vi "Main - Auto Detect Modules.vi"(8 "error in (no error)":errorcluster, 11 "Node Ptr":u64 format="%.0x") -> (0 "error out":errorcluster)   [LabVIEW 2017, in "Scan Engine Custom Device.lvlib"]
uses:
  Scan Engine Custom Device.lvlib
  <vilib>/NI Veristand/Custom Device API/Custom Device Channel.ctl
  <vilib>/NI Veristand/Custom Device API/Custom Device Channel Type.ctl
  Modules.lvlibp/RSI Module/Slot Settings.ctl
  Modules.lvlibp/RSI Module/Module Models.ctl
  Type Defs/Host - FPGAScanInterfaceMode.ctl
  Globals/String Constants.vi
  Globals/Scan Engine GUIDs.vi
  Globals/Property Strings.vi
  <vilib>/NI Veristand/Custom Device API/Set Item Property (String).vi
  Modules.lvlibp/RSI Module/Class Property Strings.vi
  Modules.lvlibp/RSI Module/RSI Module.lvclass
  Modules.lvlibp/RemIO Module/RemIO Module.lvclass
  <vilib>/NI Veristand/Custom Device API/Custom Device API.lvlib
  Modules.lvlibp
  <resource>/objmgr/ni.var.rc
panel:
  in  "Tag":string
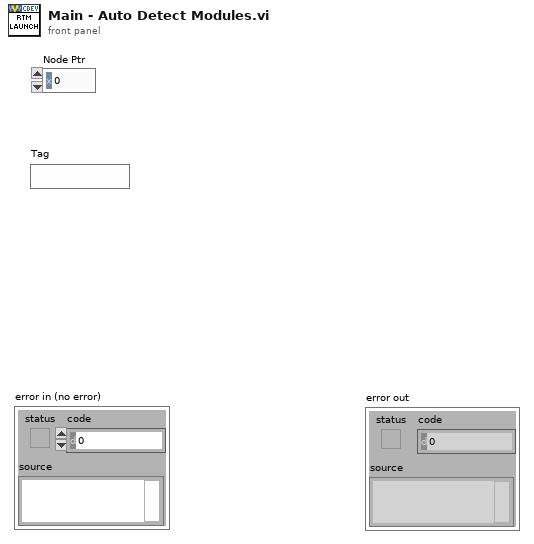
[diagram p1: front panel]
types:
  T1 = typedef "Custom Device API.lvlib/Custom Device Channel Type.ctl" = enum16{"Input", "Output"}
  T2 = typedef "Modules.lvlibp/RSI Module.lvclass/Slot Settings.ctl" = cluster{"Slot":u32, "EtherCAT?":bool}
  T3 = typedef "Modules.lvlibp/RSI Module.lvclass/Module Models.ctl" = enum16{"Empty", "NI 9201", "NI 9203", "NI 9205", "NI 9206", "NI 9207", "NI 9208", "NI 9211", "NI 9212", "NI 9213", "NI 9214", "NI 9215", "NI 9217", "NI 9219", "NI 9220", "NI 9221", "NI 9222", "NI 9223", "NI 9225", "NI 9227", "NI 9229", "NI 9233", "NI 9234", "NI 9235", "NI 9236", "NI 9237", "NI 9239", "NI 9242", "NI 9244", "NI 9263", "NI 9264", "NI 9265", "NI 9269", "NI 9375", "NI 9401", "NI 9402", "NI 9403", "NI 9411", "NI 9421", "NI 9422", "NI 9423", "NI 9425", "NI 9426", "NI 9435", "NI 9437", "NI 9472", "NI 9474", "NI 9475", "NI 9476", "NI 9477", "NI 9478", "NI 9481", "NI 9482", "NI 9485"}
  T4 = typedef "Scan Engine Custom Device.lvlib/Host - FPGAScanInterfaceMode.ctl" = enum16{"Use Current", "FPGA", "Scan Mode"}
  T5 = typedef "Custom Device API.lvlib/Custom Device Item Ref.ctl" = u64
  T6 = typedef "Custom Device API.lvlib/Custom Device Item Info.ctl" = cluster{"Name":string, "Is Channel":bool, "GUID":string, "Is Waveform":bool}
  T7 = typedef "Scan Engine Custom Device.lvlib/Host - HW Config.ctl" = cluster{"Local Chassis":T8, "Masters":T10[]}
  T8 = typedef "Scan Engine Custom Device.lvlib/Host - Local Chassis.ctl" = cluster{"Modules":T9[]}
  T9 = typedef "Scan Engine Custom Device.lvlib/Host - Module.ctl" = cluster{"IOV Ref":refnum<k21>, "Slot":u32, "Model":u32}
  T10 = typedef "Scan Engine Custom Device.lvlib/Host - Master.ctl" = cluster{"IOV Ref":refnum<k21>, "Name":string, "Master ID":u32, "Slaves":T11[]}
  T11 = typedef "Scan Engine Custom Device.lvlib/Host - Slave.ctl" = cluster{"IOV Ref":refnum<k21>, "Name":string, "Position Address":u16, "Bitfile Signature":u8[], "Modules":T9[], "ECAT Variablenobjekt":refnum<k21>[]}
  T12 = typedef "Custom Device API.lvlib/Custom Device Channel.ctl" = cluster{"Type":T1, "Units":string, "Default Value":dbl, "Faultable":bool, "Scalable":bool}
  T13 = typedef "Scan Engine Custom Device.lvlib/ECAT Channel Data Type.ctl" = enum16{"Boolean", "Fixed Point", "Int8", "Int16", "Int32", "Int64", "U32 Bit Field", "UInt8", "UInt16", "UInt32", "UInt64", "Other", "DBL"}
  T14 = typedef "Modules.lvlibp/Custom Device API.lvlib/Custom Device Item Ref.ctl" = u64
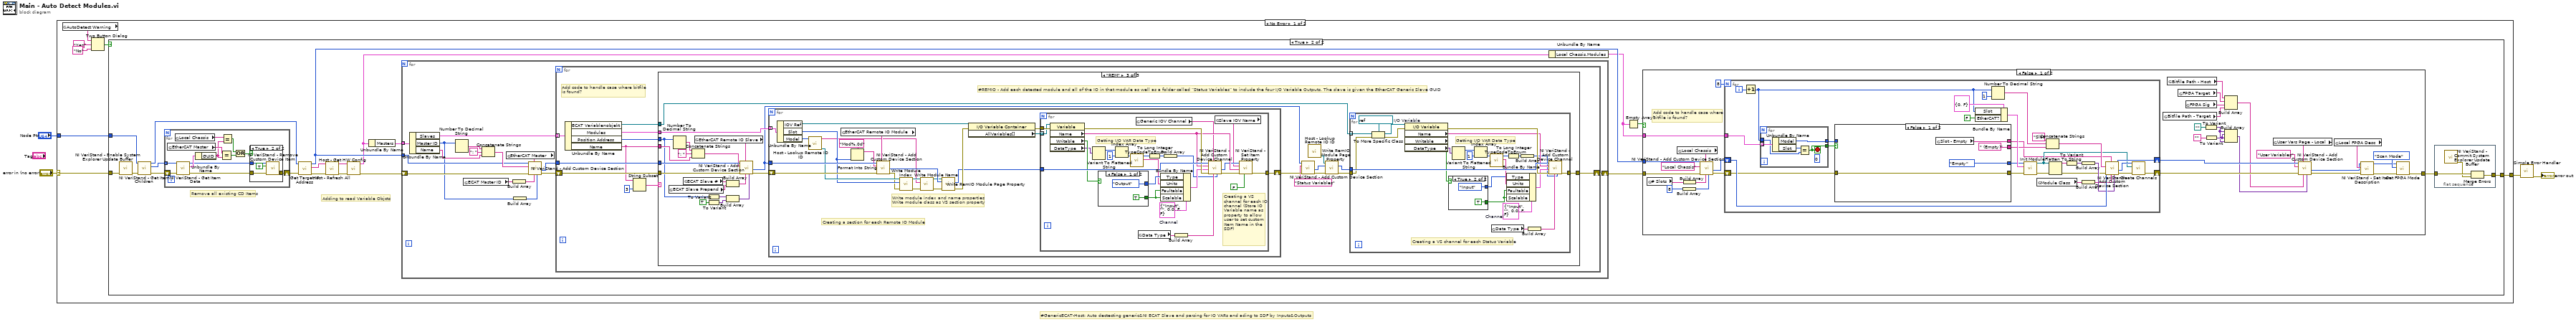
[diagram p0: block diagram]
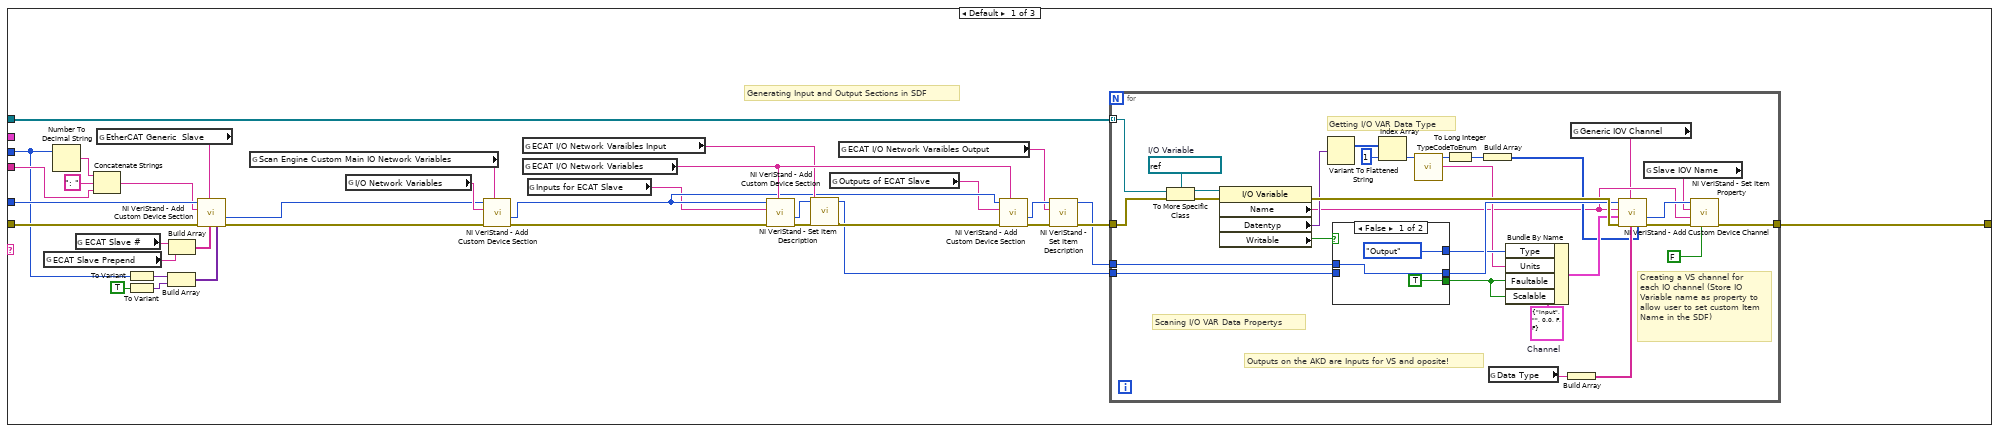
[diagram p3: hidden frame]
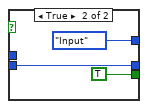
[diagram p4: hidden frame]
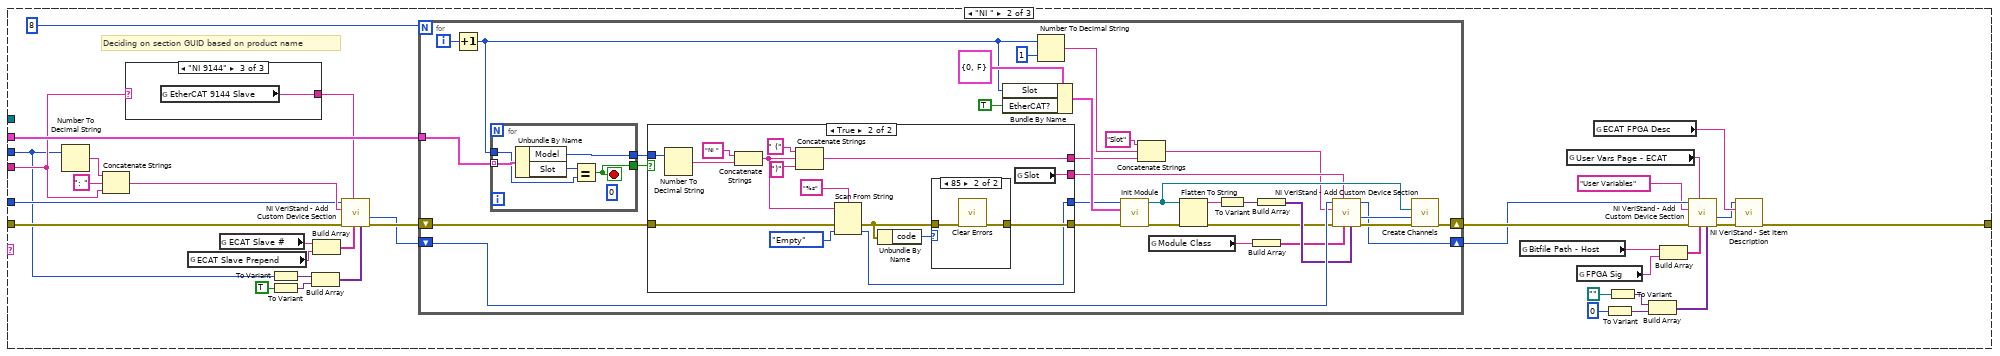
[diagram p5: hidden frame]
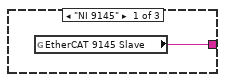
[diagram p6: hidden frame]
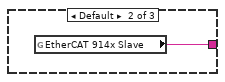
[diagram p7: hidden frame]
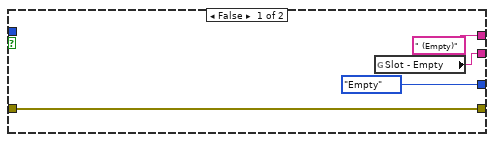
[diagram p8: hidden frame]
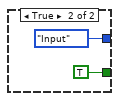
[diagram p10: hidden frame]
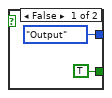
[diagram p11: hidden frame]
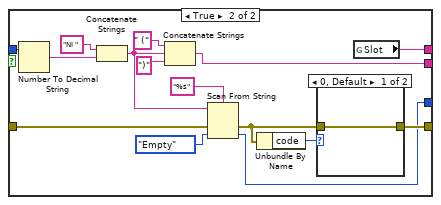
[diagram p13: hidden frame]
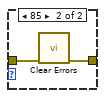
[diagram p14: hidden frame]
diagram:
  # "#GenericECAT-Host: Auto dectecting generic&NI ECAT Slave and parsing for IO VARs and ading to SDF by Inputs&Outputs"
  n1 = case shown="No Error" "error in (no error)" {
    selector: "error in (no error)" -> [w6 w444]
    tunnel: "Node Ptr" -> [w7 _]
    tunnel: [w5 w444] -> w2
    frame No Error {
      n2 = global read "String Constants.vi" "AutoDetect Warning"() -> (w8:string)
      n3 = Two Button Dialog(message=w8, 1:"No" ("F button name (\"Cancel\")"), 2:"Yes" ("T button name (\"OK\")")) -> (T button?=w11:bool)
      n4 = case shown="True" w11 {
        tunnel: w6 -> [w12 w26]
        tunnel: [w12 w14] -> w5
        tunnel: w7 -> [_ w30]
        frame False {
        }
        frame True {
          # "Adding to read Variable Objcts"
          # "Remove all existing CD Items"
          n5 = call <vilib>:"NI VeriStand - Enable System Explorer Update Buffer.vi"("error in (no error)"=w26) -> ("error out"=w25:errorcluster)  [unwired: 10 in]
          n6 = call <vilib>:"NI VeriStand - Get Item Children.vi"("error in (no error)"=w25, "Item Ref in"=w30) -> ("error out"=w31:errorcluster, "Child Refs"=w32:T5[], "Item Ref out"=w29:T5)  [unwired: 6 in, 1 out]
          n7 = for {
            tunnel: w32 -> [w347] mode=indexing
            shift-right: [w341] -> w13
            shift-left: w31 -> [w346]
            n8 = global read "Scan Engine GUIDs.vi" "EtherCAT Master"() -> (w344:string)
            n9 = global read "Scan Engine GUIDs.vi" "Local Chassis"() -> (w340:string)
            n10 = call <vilib>:"NI VeriStand - Get Item Data.vi"("error in (no error)"=w346, "Item Ref in"=w347) -> ("error out"=w342:errorcluster, "Item Info"=w345:T6, "Item Ref out"=w343:T5)  [unwired: 6 in, 1 out]
            n11 = Unbundle By Name(w345) -> ("GUID"=w339:string)
            n12 = Equal?(x=w344, y=w339) -> (x = y?=w337:bool)
            n13 = Equal?(x=w340, y=w339) -> (x = y?=w338:bool)
            n14 = Or(x=w338, y=w337) -> (x .or. y?=w336:bool)
            n15 = case shown="True" w336 {
              tunnel: w343 -> [_ w351]
              tunnel: w342 -> [w348 w352]
              tunnel: [w348 w350] -> w341
              frame False {
              }
              frame True {
                n16 = call <vilib>:"NI VeriStand - Remove Custom Device Item.vi"("error in (no error)"=w352, "Force Delete (F)"=TRUE, "Item Ref in"=w351) -> ("error out"=w350:errorcluster)  [unwired: 7 in, 1 out]
              }
            }
          }
          n17 = call "Get Target IP Address.vi"("error in"=w13, "Item Ref in"=w29) -> ("error out"=w27:errorcluster, "Target IP Address"=w28:string, "Item Ref out"=w19:T5)  [unwired: 7 in]
          n18 = call "Host - Refresh All.vi"("error in (no error)"=w27, "serverName"=w28) -> ("error out"=w24:errorcluster, "serverName"=w22:string)  [unwired: 8 in]
          n19 = call "Host - Get HW Config.vi"("error in (no error)"=w24, "serverName"=w22) -> ("error out"=w23:errorcluster, "HW Config"=w18:T7)  [unwired: 8 in]
          n20 = Unbundle By Name(w18) -> ("Masters"=w21:T10[])
          n21 = for {
            tunnel: w21 -> [w46] mode=indexing
            shift-right: [w36] -> w20
            shift-left: w23 -> [w47]
            tunnel: w19 -> [w48]
            n22 = Unbundle By Name(w46) -> ("Slaves"=w38:T11[], "Master ID"=w41:u32, "Name"=w43:string)
            n23 = Number To Decimal String(number=w41) -> (decimal integer string=w45:string)  [unwired: 1 in]
            n24 = global read "Property Strings.vi" "ECAT Master ID"() -> (w42:string)
            n25 = Concatenate Strings(w45, ": " ("string"), w43) -> (w49:string)
            n26 = global read "Scan Engine GUIDs.vi" "EtherCAT Master"() -> (w51:string)
            n27 = Build Array(w42) -> (w50:string[])
            n28 = Build Array(w41) -> (w40:u32[])
            n29 = call <vilib>:"NI VeriStand - Add Custom Device Section.vi"("Property Values"=w40, "Property names"=w50, "GUID (Default Section)"=w51, "error in (no error)"=w47, "Section Name"=w49, "Parent Ref in"=w48) -> ("error out"=w39:errorcluster, "Section Ptr"=w37:T5)  [unwired: 2 in, 2 out]
            n30 = for {
              shift-right: [w57] -> w36
              shift-left: w39 -> [w60]
              tunnel: w38 -> [w61] mode=indexing
              tunnel: w37 -> [w59]
              # "Add code to handle case where bitfile\nis found?"
              n31 = Unbundle By Name(w61) -> ("ECAT Variablenobjekt"=w55:refnum<k21>[], "Modules"=w58:T9[], "Position Address"=w53:u16, "Name"=w52:string)
              n32 = String Subset(string=w52, length (rest)=3 ("Länge (Rest)")) -> (substring=w54:string)  [unwired: 1 in]
              n33 = case shown="\"REM\"" w54 {
                tunnel: w60 -> [w79 w153 w245]
                tunnel: w58 -> [_ w152 w255]
                tunnel: [w96 w151 w252] -> w57
                tunnel: w55 -> [w97 _ w251]
                tunnel: w59 -> [w78 w138 w242]
                tunnel: w53 -> [w62 w135 w229]
                tunnel: w52 -> [w65 w137 w232]
                frame Default {
                  # "Generating Input and Output Sections in SDF"
                  n34 = global read "Property Strings.vi" "ECAT Slave Prepend"() -> (w69:string)
                  n35 = Number To Decimal String(number=w62) -> (decimal integer string=w72:string)  [unwired: 1 in]
                  n36 = global read "Property Strings.vi" "ECAT Slave #"() -> (w70:string)
                  n37 = Concatenate Strings(w72, ": " ("string"), w65) -> (w74:string)
                  n38 = global read "Scan Engine GUIDs.vi" "EtherCAT Generic  Slave"() -> (w75:string)
                  n39 = To Variant(anything=w62) -> (Variant=w68:variant)
                  n40 = To Variant(anything=TRUE) -> (Variant=w67:variant)
                  n41 = Build Array(w68, w67) -> (w64:variant[])
                  n42 = Build Array(w70, w69) -> (w71:string[])
                  n43 = call <vilib>:"NI VeriStand - Add Custom Device Section.vi"("Property Values"=w64, "Property names"=w71, "GUID (Default Section)"=w75, "error in (no error)"=w79, "Section Name"=w74, "Parent Ref in"=w78) -> ("error out"=w76:errorcluster, "Section Ptr"=w77:T5)  [unwired: 2 in, 2 out]
                  n44 = global read "Scan Engine GUIDs.vi" "Scan Engine Custom Main IO Network Variables"() -> (w89:string)
                  n45 = global read "Property Strings.vi" "I/O Network Variables"() -> (w82:string)
                  n46 = call <vilib>:"NI VeriStand - Add Custom Device Section.vi"("GUID (Default Section)"=w89, "error in (no error)"=w76, "Section Name"=w82, "Parent Ref in"=w77) -> ("error out"=w83:errorcluster, "Section Ptr"=w84:T5)  [unwired: 4 in, 2 out]
                  n47 = global read "String Constants.vi" "ECAT I/O Network Varaibles Input"() -> (w85:string)
                  n48 = global read "Scan Engine GUIDs.vi" "ECAT I/O Network Variables"() -> (w86:string)
                  n49 = global read "Property Strings.vi" "Inputs for ECAT Slave"() -> (w81:string)
                  n50 = call <vilib>:"NI VeriStand - Add Custom Device Section.vi"("GUID (Default Section)"=w86, "error in (no error)"=w83, "Section Name"=w81, "Parent Ref in"=w84) -> ("error out"=w95:errorcluster, "Section Ptr"=w88:T5)  [unwired: 4 in, 2 out]
                  n51 = call <vilib>:"NI VeriStand - Set Item Description.vi"("error in (no error)"=w95, "Description"=w85, "Item Ref in"=w88) -> ("error out"=w94:errorcluster, "Item Ref out"=w93:T5)  [unwired: 6 in, 1 out]
                  n52 = global read "Property Strings.vi" "Outputs of ECAT Slave"() -> (w80:string)
                  n53 = global read "String Constants.vi" "ECAT I/O Network Varaibles Output"() -> (w63:string)
                  n54 = call <vilib>:"NI VeriStand - Add Custom Device Section.vi"("GUID (Default Section)"=w86, "error in (no error)"=w94, "Section Name"=w80, "Parent Ref in"=w84) -> ("error out"=w92:errorcluster, "Section Ptr"=w87:T5)  [unwired: 4 in, 2 out]
                  n55 = call <vilib>:"NI VeriStand - Set Item Description.vi"("error in (no error)"=w92, "Description"=w63, "Item Ref in"=w87) -> ("error out"=w91:errorcluster, "Item Ref out"=w90:T5)  [unwired: 6 in, 1 out]
                  n56 = for {
                    tunnel: w97 -> [w110] mode=indexing
                    tunnel: [w104] -> w96
                    tunnel: w91 -> [w119]
                    tunnel: w90 -> [w118]
                    tunnel: w93 -> [w116]
                    w125 = refnum<k21> refnum  # I/O Variable
                    w127 = T12 {"Type"=enum."Input", "Units"="", "Default Value"=0.0, "Faultable"=FALSE, "Scalable"=FALSE}  # Channel
                    # "Creating a VS channel for each IO channel (Store IO Variable name as property to allow user to set custom Item Name in the SDF)"
                    # "Getting I/O VAR Data Type"
                    # "Scaning I/O VAR Data Propertys"
                    # "Outputs on the AKD are Inputs for VS and oposite!"
                    n57 = To More Specific Class(target class=w125, reference=w110, error in=w119) -> (specific class reference=w124:refnum<k21>, error out=w123:errorcluster)
                    n58 = property class="I/O Variable"(reference=w124, error in=w123) -> (error out=w128:errorcluster, "Name"=w100:string, "Datentyp"=w122:variant, "Writable"=w107:bool)  [unwired: 1 out]
                    n59 = Variant To Flattened String(Variant=w122) -> (1:w121:i16[])  [unwired: 1 out]
                    n60 = case shown="False" w107 {
                      tunnel: [Custom_Device_Channel_Type."Output" ("Type") Custom_Device_Channel_Type."Input" ("Type")] -> w114
                      tunnel: [w129 w132] -> w117
                      tunnel: w118 -> [w129 _]
                      tunnel: w116 -> [_ w132]
                      tunnel: [TRUE TRUE] -> w115
                      frame False {
                      }
                      frame True {
                      }
                    }
                    n61 = Index Array(array=w121, index=1) -> (element=w112:i16)
                    n62 = call "TypeCodeToEnum.vi"("Type Code (numbers in hexadecimal)"=w112) -> (2:"UDV Data Type"=w113:string, 3:"UDV Data Type"=w111:T13)  [unwired: 9 in]
                    n63 = To Long Integer(number=w111) -> (32bit integer=w106:i32)
                    n64 = Build Array(w106) -> (w102:i32[])
                    n65 = global read "Property Strings.vi" "Data Type"() -> (w109:string)
                    n66 = Bundle By Name(cluster=w127, "Type"=w114, "Units"=w113, "Faultable"=w115, "Scalable"=w115) -> (w126:T12)
                    n67 = Build Array(w109) -> (w108:string[])
                    n68 = global read "Scan Engine GUIDs.vi" "Generic IOV Channel"() -> (w99:string)
                    n69 = call <vilib>:"NI VeriStand - Add Custom Device Channel.vi"("Property Values"=w102, "Property names"=w108, "GUID (Default Channel)"=w99, "error in (no error)"=w128, "Channel"=w126, "Channel Name"=w100, "Parent Ref in"=w117) -> ("error out"=w105:errorcluster, "Channel Ref"=w103:T5)  [unwired: 1 in, 2 out]
                    n70 = global read "Property Strings.vi" "Slave IOV Name"() -> (w101:string)
                    n71 = call-poly <vilib>:"NI VeriStand - Set Item Property.vi"("Binary String (T)"=FALSE, "error in (no error)"=w105, "Value"=w100, "Property Name"=w101, "Item Ref in"=w103) -> ("error out"=w104:errorcluster)  [unwired: 4 in, 2 out]
                  }
                }
                frame "NI " {
                  # "Deciding on section GUID based on product name"
                  n72 = Number To Decimal String(number=w135) -> (decimal integer string=w149:string)  [unwired: 1 in]
                  n73 = Concatenate Strings(w149, ": " ("string"), w137) -> (w147:string)
                  n74 = case shown="\"NI 9144\"" w137 {
                    tunnel: [w169 w170 w171] -> w136
                    frame "NI 9145" {
                      n75 = global read "Scan Engine GUIDs.vi" "EtherCAT 9145 Slave"() -> (w169:string)
                    }
                    frame Default {
                      n76 = global read "Scan Engine GUIDs.vi" "EtherCAT 914x Slave"() -> (w170:string)
                    }
                    frame "NI 9144" {
                      n77 = global read "Scan Engine GUIDs.vi" "EtherCAT 9144 Slave"() -> (w171:string)
                    }
                  }
                  n78 = global read "Property Strings.vi" "ECAT Slave Prepend"() -> (w145:string)
                  n79 = global read "Property Strings.vi" "ECAT Slave #"() -> (w144:string)
                  n80 = To Variant(anything=w135) -> (Variant=w146:variant)
                  n81 = To Variant(anything=TRUE) -> (Variant=w140:variant)
                  n82 = Build Array(w146, w140) -> (w142:variant[])
                  n83 = Build Array(w144, w145) -> (w143:string[])
                  n84 = call <vilib>:"NI VeriStand - Add Custom Device Section.vi"("Property Values"=w142, "Property names"=w143, "GUID (Default Section)"=w136, "Section Name"=w147, "Parent Ref in"=w138) -> ("Section Ptr"=w139:T5)  [unwired: 3 in, 3 out]
                  n85 = for {
                    N: 8 -> [_]
                    shift-right: [w175] -> w164
                    shift-left: w153 -> [w181]
                    shift-right: [w173] -> w163
                    shift-left: w139 -> [w201]
                    tunnel: w152 -> [w186]
                    i -> [w198]
                    n86 = Increment(x=w198) -> (x+1=w185:i32)
                    n87 = for {
                      tunnel: w186 -> [w228] mode=indexing
                      tunnel: w185 -> [w226]
                      tunnel: [w225] -> w184
                      tunnel: [w224] -> w179
                      stop <- w225 stop-if-true
                      (unwired) u32 0 ("Model")
                      n88 = Unbundle By Name(w228) -> ("Model"=w224:u32, "Slot"=w227:u32)
                      n89 = Equal?(x=w227, y=w226) -> (x = y?=w225:bool)
                    }
                    n90 = case shown="True" w184 {
                      tunnel: [" (Empty)" ("Section Name") w207] -> w183
                      tunnel: [Module_Models."Empty" ("Module") w214] -> w182
                      tunnel: w181 -> [w203 w215]
                      tunnel: [w203 w216] -> w180
                      tunnel: w179 -> [_ w213]
                      tunnel: [w202 w206] -> w174
                      frame False {
                        n91 = global read "Scan Engine GUIDs.vi" "Slot - Empty"() -> (w202:string)
                      }
                      frame True {
                        n92 = Number To Decimal String(number=w213) -> (decimal integer string=w212:string)  [unwired: 1 in]
                        n93 = Concatenate Strings("NI " ("string"), w212) -> (w210:string)
                        n94 = Concatenate Strings(" (" ("string"), w210, ")" ("string")) -> (w207:string)
                        n95 = Scan From String(format string="%s", input string=w210, error in=w215, default 1=Module_Models."Empty" ("Module")) -> (error out=w217:errorcluster, output 1=w214:T3)  [unwired: 1 in, 2 out]
                        n96 = Unbundle By Name(w217) -> ("code"=w218:i32)
                        n97 = case shown="85" w218 {
                          tunnel: [w221 w222] -> w216
                          tunnel: w217 -> [w221 w223]
                          frame 0, Default {
                          }
                          frame 85 {
                            n98 = call <vilib>:"Clear Errors.vi"("error in (no error)"=w223) -> ("error out"=w222:errorcluster)  [unwired: 5 in, 1 out]
                          }
                        }
                        n99 = global read "Scan Engine GUIDs.vi" "Slot"() -> (w206:string)
                      }
                    }
                    n100 = Bundle By Name(cluster=T2 {"Slot"=0, "EtherCAT?"=FALSE} ("Slot Settings"), "Slot"=w185, "EtherCAT?"=TRUE) -> (w195:T2)
                    n101 = Number To Decimal String(number=w185, width (-)=i16 1) -> (decimal integer string=w200:string)
                    n102 = call "Init Module.vi"("error in (no error)"=w180, "Slot Settings"=w195, "Module Model"=w182) -> ("error out"=w190:errorcluster, "RSI Module out"=w176:refnum<class "RSI Module.lvclass">)  [unwired: 7 in]
                    n103 = Concatenate Strings("Slot" ("string"), w200, w183) -> (w172:string)
                    n104 = global read "Class Property Strings.vi" "Module Class"() -> (w188:string)
                    n105 = Flatten To String(anything=w176, error in (no error)=w190) -> (data string=w191:string, error out=w189:errorcluster)  [unwired: 2 in, 1 out]
                    n106 = To Variant(anything=w191) -> (Variant=w196:variant)
                    n107 = Build Array(w188) -> (w192:string[])
                    n108 = Build Array(w196) -> (w197:variant[])
                    n109 = call <vilib>:"NI VeriStand - Add Custom Device Section.vi"("Property Values"=w197, "Property names"=w192, "GUID (Default Section)"=w174, "error in (no error)"=w189, "Section Name"=w172, "Parent Ref in"=w201) -> ("error out"=w177:errorcluster, "Section Ptr"=w178:T5, "Parent Ref out"=w173:T5)  [unwired: 2 in, 1 out]
                    n110 = call-dynamic "Create Channels.vi"("error in (no error)"=w177, "RSI Module in"=w176, "Parent Ref in"=w178) -> ("error out"=w175:errorcluster)  [unwired: 6 in, 2 out]
                  }
                  n111 = global read "Property Strings.vi" "Bitfile Path - Host"() -> (w155:string)
                  n112 = global read "Scan Engine GUIDs.vi" "User Vars Page - ECAT"() -> (w166:string)
                  n113 = global read "Property Strings.vi" "FPGA Sig"() -> (w154:string)
                  n114 = global read "String Constants.vi" "ECAT FPGA Desc"() -> (w165:string)
                  n115 = To Variant(anything=u32 0 ("ModuleIdent (ECAT)")) -> (Variant=w156:variant)
                  n116 = To Variant(anything=path "") -> (Variant=w157:variant)
                  n117 = Build Array(w157, w156) -> (w167:variant[])
                  n118 = Build Array(w155, w154) -> (w168:string[])
                  n119 = call <vilib>:"NI VeriStand - Add Custom Device Section.vi"("Property Values"=w167, "Property names"=w168, "GUID (Default Section)"=w166, "error in (no error)"=w164, "Section Name"="User Variables", "Parent Ref in"=w163) -> ("error out"=w160:errorcluster, "Section Ptr"=w161:T5)  [unwired: 2 in, 2 out]
                  n120 = call <vilib>:"NI VeriStand - Set Item Description.vi"("error in (no error)"=w160, "Description"=w165, "Item Ref in"=w161) -> ("error out"=w151:errorcluster)  [unwired: 6 in, 2 out]
                }
                frame "REM" {
                  # "#REMIO - Add each detected module and all of the IO in that module as well as a folder called “Status Variables” to include the four I/O Variable Outputs. The slave is given the EtherCAT Generic Slave GUID"
                  n121 = global read "Property Strings.vi" "ECAT Slave Prepend"() -> (w236:string)
                  n122 = Number To Decimal String(number=w229) -> (decimal integer string=w240:string)  [unwired: 1 in]
                  n123 = global read "Property Strings.vi" "ECAT Slave #"() -> (w235:string)
                  n124 = Concatenate Strings(w240, ": " ("string"), w232) -> (w238:string)
                  n125 = global read "Scan Engine GUIDs.vi" "EtherCAT Remote IO Slave"() -> (w241:string)
                  n126 = To Variant(anything=w229) -> (Variant=w237:variant)
                  n127 = To Variant(anything=TRUE) -> (Variant=w230:variant)
                  n128 = Build Array(w237, w230) -> (w233:variant[])
                  n129 = Build Array(w235, w236) -> (w234:string[])
                  n130 = call <vilib>:"NI VeriStand - Add Custom Device Section.vi"("Property Values"=w233, "Property names"=w234, "GUID (Default Section)"=w241, "error in (no error)"=w245, "Section Name"=w238, "Parent Ref in"=w242) -> ("error out"=w244:errorcluster, "Section Ptr"=w243:T5)  [unwired: 2 in, 2 out]
                  n131 = for {
                    shift-right: [w271] -> w254
                    shift-left: w244 -> [w277]
                    tunnel: w243 -> [w276]
                    tunnel: w255 -> [w275] mode=indexing
                    # "Write module index and name properties\nWrite module class as VS section property"
                    # "Creating a section for each Remote IO Module"
                    n132 = Unbundle By Name(w275) -> ("IOV Ref"=w274:refnum<k21>, "Slot"=w267:u32, "Model"=w270:u32)
                    n133 = call "Host - Lookup Remote IO ID.vi"("Module ID"=w270) -> ("RemIO Module Out"=w268:refnum<class "RemIO Module.lvclass">, "Module Name"=w256:string)  [unwired: 9 in]
                    n134 = global read "Scan Engine GUIDs.vi" "EtherCAT Remote IO Module"() -> (w266:string)
                    n135 = Format Into String(format string="Mod%.0d", w267) -> (resulting string=w262:string)  [unwired: 2 in, 1 out]
                    n136 = call <vilib>:"NI VeriStand - Add Custom Device Section.vi"("GUID (Default Section)"=w266, "error in (no error)"=w277, "Section Name"=w262, "Parent Ref in"=w276) -> ("error out"=w264:errorcluster, "Section Ptr"=w265:T5)  [unwired: 4 in, 2 out]
                    n137 = call-dynamic "Write Module Index.vi"("error in (no error)"=w264, "Module Index"=w267, "RemIO Module in"=w268) -> ("error out"=w259:errorcluster, "RemIO Module out"=w260:refnum<class "RemIO Module.lvclass">)  [unwired: 7 in]
                    n138 = call-dynamic "Write Module Name.vi"("error in (no error)"=w259, "Module Name"=w256, "RemIO Module in"=w260) -> ("error out"=w258:errorcluster, "RemIO Module out"=w257:refnum<class "RemIO Module.lvclass">)  [unwired: 7 in]
                    n139 = call "Write RemIO Module Page Property.vi"("error in (no error)"=w258, "Node Ptr In"=w265, "RemIO Module"=w257) -> ("error out"=w269:errorcluster, "Node Ptr Out"=w263:T14)  [unwired: 6 in, 1 out]
                    n140 = property class="I/O Variable Container"(reference=w274, error in=w269) -> (error out=w272:errorcluster, "AllVariables[]"=w273:refnum<k21>[])  [unwired: 1 out]
                    n141 = for {
                      tunnel: w273 -> [w301] mode=indexing
                      tunnel: w263 -> [w303]
                      tunnel: w272 -> [w302]
                      tunnel: [w284] -> w271
                      w299 = T12 {"Type"=enum."Input", "Units"="", "Default Value"=0.0, "Faultable"=FALSE, "Scalable"=FALSE}  # Channel
                      # "Getting I/O VAR Data Type"
                      # "Creating a VS channel for each IO channel (Store IO Variable name as property to allow user to set custom Item Name in the SDF)"
                      n142 = property class="Variable"(reference=w301, error in=w302) -> (error out=w300:errorcluster, "Name"=w283:string, "Writable"=w298:bool, "DataType"=w293:variant)  [unwired: 1 out]
                      n143 = Variant To Flattened String(Variant=w293) -> (1:w294:i16[])  [unwired: 1 out]
                      n144 = case shown="False" w298 {
                        tunnel: [TRUE TRUE] -> w297
                        tunnel: [Custom_Device_Channel_Type."Output" ("Type") Custom_Device_Channel_Type."Input" ("Type")] -> w288
                        frame False {
                        }
                        frame True {
                        }
                      }
                      n145 = Index Array(array=w294, index=1) -> (element=w296:i16)
                      n146 = call "TypeCodeToEnum.vi"("Type Code (numbers in hexadecimal)"=w296) -> (2:"UDV Data Type"=w280:string, 3:"UDV Data Type"=w291:T13)  [unwired: 9 in]
                      n147 = global read "Scan Engine GUIDs.vi" "Generic IOV Channel"() -> (w279:string)
                      n148 = global read "Property Strings.vi" "Data Type"() -> (w290:string)
                      n149 = To Long Integer(number=w291) -> (32bit integer=w287:i32)
                      n150 = Bundle By Name(cluster=w299, "Type"=w288, "Units"=w280, "Faultable"=w297, "Scalable"=w297) -> (w292:T12)
                      n151 = Build Array(w287) -> (w286:i32[])
                      n152 = Build Array(w290) -> (w289:string[])
                      n153 = call <vilib>:"NI VeriStand - Add Custom Device Channel.vi"("Property Values"=w286, "Property names"=w289, "GUID (Default Channel)"=w279, "error in (no error)"=w300, "Channel"=w292, "Channel Name"=w283, "Parent Ref in"=w303) -> ("error out"=w285:errorcluster, "Channel Ref"=w282:T5)  [unwired: 1 in, 2 out]
                      n154 = global read "Property Strings.vi" "Slave IOV Name"() -> (w281:string)
                      n155 = call-poly <vilib>:"NI VeriStand - Set Item Property.vi"("Binary String (T)"=FALSE, "error in (no error)"=w285, "Value"=w283, "Property Name"=w281, "Item Ref in"=w282) -> ("error out"=w284:errorcluster)  [unwired: 4 in, 2 out]
                    }
                  }
                  n156 = call <vilib>:"NI VeriStand - Add Custom Device Section.vi"("error in (no error)"=w254, "Section Name"="Status Variables", "Parent Ref in"=w243) -> ("error out"=w250:errorcluster, "Section Ptr"=w248:T5)  [unwired: 5 in, 2 out]
                  n157 = call "Host - Lookup Remote IO ID.vi"() -> ("RemIO Module Out"=w246:refnum<class "RemIO Module.lvclass">)  [unwired: 10 in, 1 out]
                  n158 = call "Write RemIO Module Page Property.vi"("error in (no error)"=w250, "Node Ptr In"=w248, "RemIO Module"=w246) -> ("error out"=w249:errorcluster, "Node Ptr Out"=w247:T14)  [unwired: 6 in, 1 out]
                  n159 = for {
                    tunnel: w251 -> [w330] mode=indexing
                    tunnel: w247 -> [w331]
                    tunnel: [w310] -> w252
                    tunnel: w249 -> [w308]
                    w317 = refnum<k21> refnum  # I/O Variable
                    w327 = T12 {"Type"=enum."Input", "Units"="", "Default Value"=0.0, "Faultable"=FALSE, "Scalable"=FALSE}  # Channel
                    # "Creating a VS channel for each Status Variable"
                    # "Getting I/O VAR Data Type"
                    n160 = To More Specific Class(target class=w317, reference=w330, error in=w308) -> (specific class reference=w318:refnum<k21>, error out=w319:errorcluster)
                    n161 = property class="I/O Variable"(reference=w318, error in=w319) -> (error out=w329:errorcluster, "Name"=w328:string, "Writable"=w326:bool, "DataType"=w321:variant)  [unwired: 1 out]
                    n162 = case shown="True" w326 {
                      tunnel: [Custom_Device_Channel_Type."Output" ("Type") Custom_Device_Channel_Type."Input" ("Type")] -> w309
                      tunnel: [TRUE TRUE] -> w325
                      frame False {
                      }
                      frame True {
                      }
                    }
                    n163 = Variant To Flattened String(Variant=w321) -> (1:w322:i16[])  [unwired: 1 out]
                    n164 = Index Array(array=w322, index=1) -> (element=w324:i16)
                    n165 = call "TypeCodeToEnum.vi"("Type Code (numbers in hexadecimal)"=w324) -> (2:"UDV Data Type"=w320:string, 3:"UDV Data Type"=w312:T13)  [unwired: 9 in]
                    n166 = global read "Property Strings.vi" "Data Type"() -> (w315:string)
                    n167 = Bundle By Name(cluster=w327, "Type"=w309, "Units"=w320, "Faultable"=w325, "Scalable"=w325) -> (w316:T12)
                    n168 = To Long Integer(number=w312) -> (32bit integer=w313:i32)
                    n169 = Build Array(w313) -> (w311:i32[])
                    n170 = Build Array(w315) -> (w314:string[])
                    n171 = call <vilib>:"NI VeriStand - Add Custom Device Channel.vi"("Property Values"=w311, "Property names"=w314, "error in (no error)"=w329, "Channel"=w316, "Channel Name"=w328, "Parent Ref in"=w331) -> ("error out"=w310:errorcluster)  [unwired: 2 in, 3 out]
                  }
                }
              }
            }
          }
          n172 = Unbundle By Name(w18) -> ("Local Chassis.Modules"=w17:T9[])
          n173 = Empty Array?(array=w17) -> (empty?=w16:bool)
          n174 = case shown="False" w16 {
            tunnel: w20 -> [w385 w443]
            tunnel: w19 -> [w384 _]
            tunnel: w17 -> [w383 _]
            tunnel: [w354 w443] -> w15
            frame False {
              # "Add code to handle case where\nbitfile is found?"
              n175 = global read "Property Strings.vi" "# Slots"() -> (w381:string)
              n176 = global read "Scan Engine GUIDs.vi" "Local Chassis"() -> (w382:string)
              n177 = Build Array(8 ("# Slots")) -> (w379:i32[])
              n178 = Build Array(w381) -> (w380:string[])
              n179 = call <vilib>:"NI VeriStand - Add Custom Device Section.vi"("Property Values"=w379, "Property names"=w380, "GUID (Default Section)"=w382, "error in (no error)"=w385, "Section Name"="Local Chassis", "Parent Ref in"=w384) -> ("error out"=w376:errorcluster, "Section Ptr"=w374:T5)  [unwired: 2 in, 2 out]
              n180 = for {
                N: 8 -> [_]
                shift-right: [w387] -> w378
                shift-left: w376 -> [w393]
                shift-right: [w410] -> w377
                shift-left: w374 -> [w415]
                tunnel: w383 -> [w398]
                i -> [w412]
                n181 = Increment(x=w412) -> (x+1=w397:i32)
                n182 = for {
                  tunnel: w398 -> [w442] mode=indexing
                  tunnel: w397 -> [w440]
                  tunnel: [w439] -> w396
                  tunnel: [w438] -> w391
                  stop <- w439 stop-if-true
                  (unwired) u32 0 ("Model")
                  n183 = Unbundle By Name(w442) -> ("Model"=w438:u32, "Slot"=w441:u32)
                  n184 = Equal?(x=w441, y=w440) -> (x = y?=w439:bool)
                }
                n185 = case shown="False" w396 {
                  tunnel: [" (Empty)" ("Section Name") w421] -> w395
                  tunnel: [Module_Models."Empty" ("Module") w428] -> w394
                  tunnel: w393 -> [w417 w429]
                  tunnel: [w417 w430] -> w392
                  tunnel: w391 -> [_ w427]
                  tunnel: [w416 w420] -> w386
                  frame False {
                    n186 = global read "Scan Engine GUIDs.vi" "Slot - Empty"() -> (w416:string)
                  }
                  frame True {
                    n187 = Number To Decimal String(number=w427) -> (decimal integer string=w426:string)  [unwired: 1 in]
                    n188 = Concatenate Strings("NI " ("string"), w426) -> (w424:string)
                    n189 = Concatenate Strings(" (" ("string"), w424, ")" ("string")) -> (w421:string)
                    n190 = Scan From String(format string="%s", input string=w424, error in=w429, default 1=Module_Models."Empty" ("Module")) -> (error out=w431:errorcluster, output 1=w428:T3)  [unwired: 1 in, 2 out]
                    n191 = Unbundle By Name(w431) -> ("code"=w432:i32)
                    n192 = case shown="0, Default" w432 {
                      tunnel: [w435 w436] -> w430
                      tunnel: w431 -> [w435 w437]
                      frame 0, Default {
                      }
                      frame 85 {
                        n193 = call <vilib>:"Clear Errors.vi"("error in (no error)"=w437) -> ("error out"=w436:errorcluster)  [unwired: 5 in, 1 out]
                      }
                    }
                    n194 = global read "Scan Engine GUIDs.vi" "Slot"() -> (w420:string)
                  }
                }
                n195 = Bundle By Name(cluster=T2 {"Slot"=0, "EtherCAT?"=FALSE} ("Slot Settings"), "Slot"=w397, "EtherCAT?"=FALSE) -> (w407:T2)
                n196 = Number To Decimal String(number=w397, width (-)=i16 1) -> (decimal integer string=w414:string)
                n197 = call "Init Module.vi"("error in (no error)"=w392, "Slot Settings"=w407, "Module Model"=w394) -> ("error out"=w402:errorcluster, "RSI Module out"=w388:refnum<class "RSI Module.lvclass">)  [unwired: 7 in]
                n198 = global read "Class Property Strings.vi" "Module Class"() -> (w400:string)
                n199 = Concatenate Strings("Slot" ("string"), w414, w395) -> (w411:string)
                n200 = Flatten To String(anything=w388, error in (no error)=w402) -> (data string=w403:string, error out=w401:errorcluster)  [unwired: 2 in, 1 out]
                n201 = To Variant(anything=w403) -> (Variant=w408:variant)
                n202 = Build Array(w408) -> (w409:variant[])
                n203 = Build Array(w400) -> (w404:string[])
                n204 = call <vilib>:"NI VeriStand - Add Custom Device Section.vi"("Property Values"=w409, "Property names"=w404, "GUID (Default Section)"=w386, "error in (no error)"=w401, "Section Name"=w411, "Parent Ref in"=w415) -> ("error out"=w389:errorcluster, "Section Ptr"=w390:T5, "Parent Ref out"=w410:T5)  [unwired: 2 in, 1 out]
                n205 = call-dynamic "Create Channels.vi"("error in (no error)"=w389, "RSI Module in"=w388, "Parent Ref in"=w390) -> ("error out"=w387:errorcluster)  [unwired: 6 in, 2 out]
              }
              n206 = global read "Property Strings.vi" "Bitfile Path - Target"() -> (w368:string)
              n207 = global read "Property Strings.vi" "Bitfile Path - Host"() -> (w365:string)
              n208 = global read "Property Strings.vi" "FPGA Target"() -> (w366:string)
              n209 = global read "Property Strings.vi" "FPGA Sig"() -> (w367:string)
              n210 = To Variant(anything=path "") -> (Variant=w369:variant)
              n211 = To Variant(anything="") -> (Variant=w371:variant)
              n212 = Build Array(w365, w366, w367, w368) -> (w363:string[])
              n213 = Build Array(w369, w371, w371, w369) -> (w362:variant[])
              n214 = global read "Scan Engine GUIDs.vi" "User Vars Page - Local"() -> (w361:string)
              n215 = call <vilib>:"NI VeriStand - Add Custom Device Section.vi"("Property Values"=w362, "Property names"=w363, "GUID (Default Section)"=w361, "error in (no error)"=w378, "Section Name"="User Variables", "Parent Ref in"=w377) -> ("error out"=w357:errorcluster, "Section Ptr"=w358:T5)  [unwired: 2 in, 2 out]
              n216 = global read "String Constants.vi" "Local FPGA Desc"() -> (w360:string)
              n217 = call <vilib>:"NI VeriStand - Set Item Description.vi"("error in (no error)"=w357, "Description"=w360, "Item Ref in"=w358) -> ("error out"=w355:errorcluster, "Item Ref out"=w353:T5)  [unwired: 6 in, 1 out]
              n218 = call "Set FPGA Mode.vi"("error in (no error)"=w355, "FPGAScanInterfaceMode"=Host_-_FPGAScanInterfaceMode."Scan Mode", "Item Ref in"=w353) -> ("error out"=w354:errorcluster)  [unwired: 7 in, 1 out]
            }
            frame True {
            }
          }
          n219 = flat-sequence {
            tunnel: w15 -> [w35]
            tunnel: [w33] -> w14
            frame #0 {
              n220 = call <vilib>:"NI VeriStand - Commit System Explorer Update Buffer.vi"() -> ("error out"=w34:errorcluster)  [unwired: 11 in]
              n221 = Merge Errors(w35, w34) -> (w33:errorcluster)
            }
          }
        }
      }
    }
    frame Error {
    }
  }
  n222 = call <vilib>:"Simple Error Handler.vi"("error in (no error)"=w2) -> ("error out"=→"error out":errorcluster)  [unwired: 4 in, 4 out]
